vi "DNVideoX.vi"() -> ()   [LabVIEW 2015]
doc: "wdyjz@126.com\n完全访问USB cam， IP 网络照相机，TV tuner， DV 摄像机， PCI采集卡，fire-wire 或其他WDM兼容设备 \n支持多种视频输入"
panel:
  in  "Stop Capture":bool
  in  "StartCapture":bool
  in  "LEDOFF":bool
  in  "LED2":bool
  in  "LED1":bool
  in  "DNVideoX":refnum<k7>(container)
  out "Saved successfully":bool
  in  "Show Video Source Dialog":bool
  in  "Show Video Format Dialog":bool
  out "Camera count list":string[](array[string])
  out "Camera count":i32
  in  "Save Image":bool
  in  "氨ゎ":bool
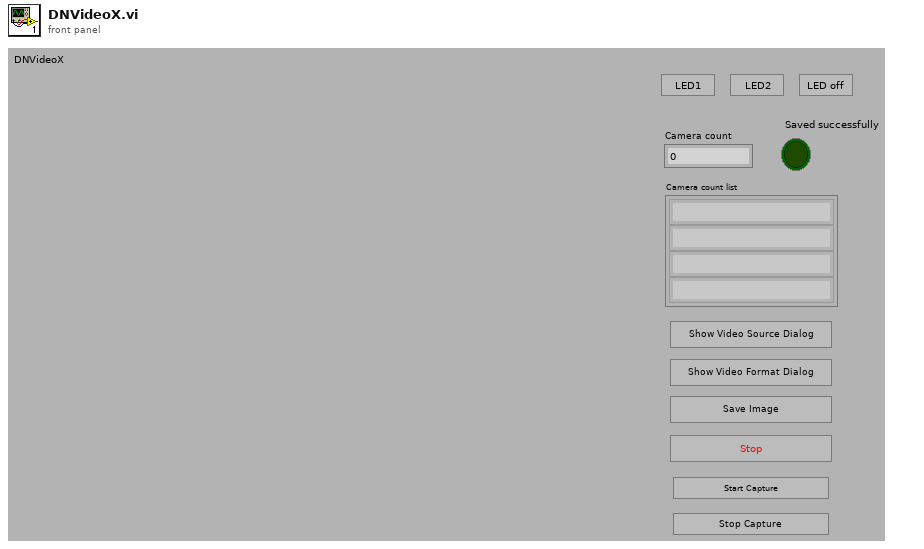
[diagram p1: front panel]
types:
  T1 = typedef "LVDateTimeRec.ctl" = cluster{"秒数的小数部分":dbl, "秒":i32, "分":i32, "小时":i32, "日":i32, "月":i32, "年":i32, "天数（周）":i32, "天数（年）":i32, "DST":i32}
  T2 = cluster{"秒数的小数部分":string, "秒":string, "分":string, "小时":string, "日":string, "月":string, "年":string, "天数（周）":string, "天数（年）":string, "DST":string}
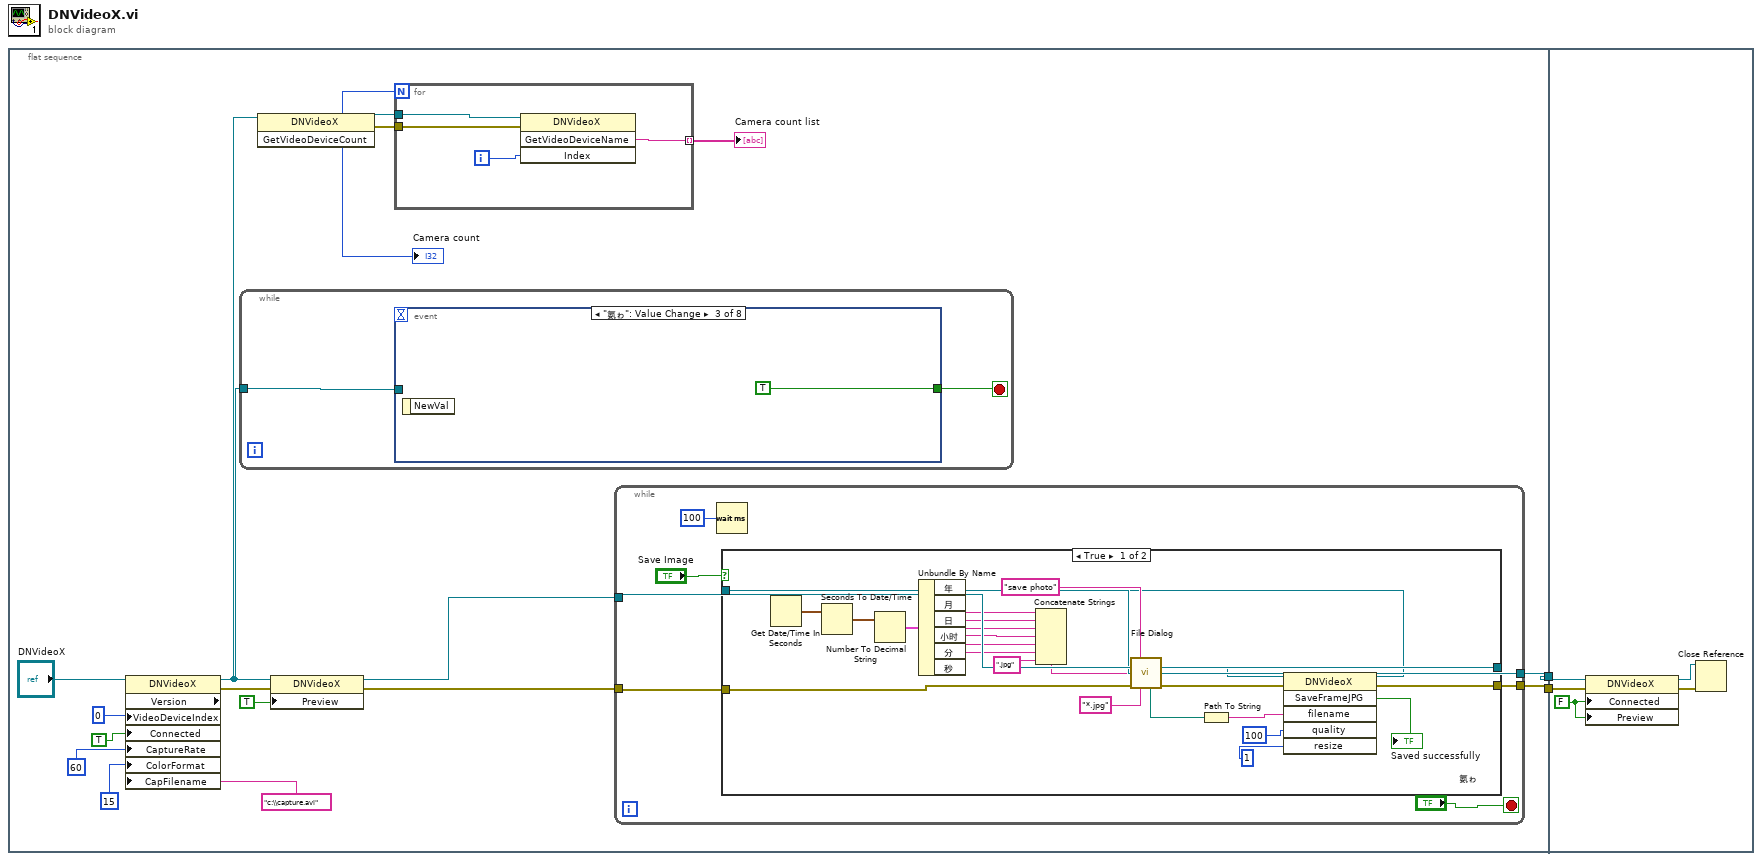
[diagram p0: block diagram]
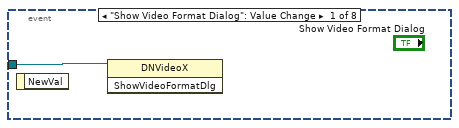
[diagram p2: hidden frame]
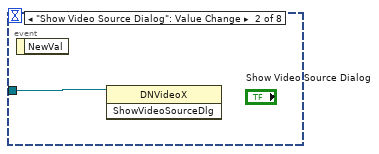
[diagram p3: hidden frame]
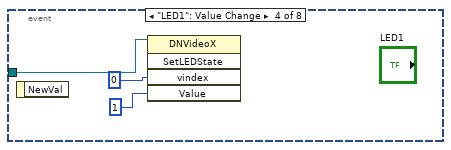
[diagram p4: hidden frame]
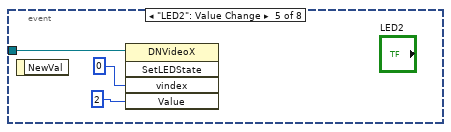
[diagram p5: hidden frame]
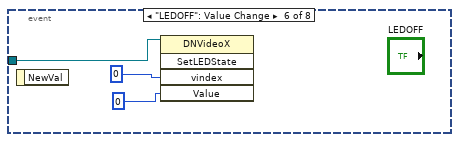
[diagram p6: hidden frame]
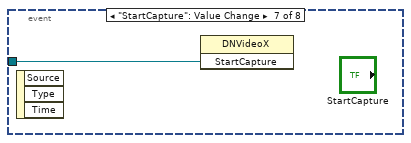
[diagram p7: hidden frame]
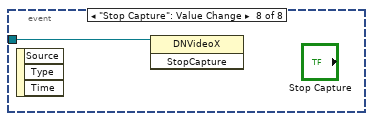
[diagram p8: hidden frame]
diagram:
  n1 = flat-sequence {
    tunnel: [w16] -> w2
    tunnel: [w9] -> w1
    tunnel: w2 -> [w76]
    tunnel: w1 -> [w72]
    frame #0 {
      n2 = property class="DNVideoX" props=["Version", "VideoDeviceIndex", "Connected", "CaptureRate", "ColorFormat", "CapFilename"](reference="DNVideoX", "VideoDeviceIndex"=0, "Connected"=TRUE, "CaptureRate"=60 ("VideoDeviceIndex"), "ColorFormat"=15 ("VideoDeviceIndex"), "CapFilename"="c:\\capture.avi" ("default name")) -> (reference out=w7:refnum<k7>, error out=w14:errorcluster)  [unwired: 1 in, 1 out]
      n3 = while {
        tunnel: w7 -> [w21]
        stop <- w20 stop-if-true
        n4 = event shown="[2] \"氨ゎ\": Value Change" {
          selector: _ -> [_ _ _ _ _ _ _ _]
          dyn-events: _ -> [_ _ _ _ _ _ _ _]
          timeout: _ -> [_ _ _ _ _ _ _ _]
          tunnel: w21 -> [w22 w23 _ w27 w30 w33 w34 w35]
          tunnel: [_ _ TRUE _ _ _ _ _] -> w20
          event "Show Video Format Dialog": Value Change {
            n5 = event-data() -> ()  [unwired: 2 out]
            n6 = invoke class="DNVideoX" method="ShowVideoFormatDlg"(reference=w22) -> ()  [unwired: 2 in, 3 out]
          }
          event "Show Video Source Dialog": Value Change {
            n7 = event-data() -> ()  [unwired: 2 out]
            n8 = invoke class="DNVideoX" method="ShowVideoSourceDlg"(reference=w23) -> ()  [unwired: 2 in, 3 out]
          }
          event "氨ゎ": Value Change {
            n9 = event-data() -> ()  [unwired: 2 out]
          }
          event "LED1": Value Change {
            n10 = event-data() -> ()  [unwired: 2 out]
            n11 = invoke class="DNVideoX" method="SetLEDState"(reference=w27, "vindex"=0, "Value"=1) -> ()  [unwired: 2 in, 5 out]
          }
          event "LED2": Value Change {
            n12 = event-data() -> ()  [unwired: 2 out]
            n13 = invoke class="DNVideoX" method="SetLEDState"(reference=w30, "vindex"=0, "Value"=2) -> ()  [unwired: 2 in, 5 out]
          }
          event "LEDOFF": Value Change {
            n14 = event-data() -> ()  [unwired: 2 out]
            n15 = invoke class="DNVideoX" method="SetLEDState"(reference=w33, "vindex"=0, "Value"=0) -> ()  [unwired: 2 in, 5 out]
          }
          event "StartCapture": Value Change {
            n16 = event-data() -> ()  [unwired: 4 out]
            n17 = invoke class="DNVideoX" method="StartCapture"(reference=w34) -> ()  [unwired: 2 in, 3 out]
          }
          event "Stop Capture": Value Change {
            n18 = event-data() -> ()  [unwired: 4 out]
            n19 = invoke class="DNVideoX" method="StopCapture"(reference=w35) -> ()  [unwired: 2 in, 3 out]
          }
        }
      }
      n20 = invoke class="DNVideoX" method="GetVideoDeviceCount"(reference=w7) -> (reference out=w10:refnum<k7>, error out=w12:errorcluster, "GetVideoDeviceCount"=w11:i32)  [unwired: 2 in]
      "Camera count" <- w11
      n21 = property class="DNVideoX"(reference=w7, error in=w14, "Preview"=TRUE) -> (reference out=w6:refnum<k7>, error out=w13:errorcluster)
      n22 = for {
        N: w11 -> [_]
        tunnel: [w36] -> w19 mode=indexing
        tunnel: w12 -> [w38]
        tunnel: w10 -> [w37]
        i -> [w39]
        n23 = invoke class="DNVideoX" method="GetVideoDeviceName"(reference=w37, error in=w38, "Index"=w39) -> ("GetVideoDeviceName"=w36:string)  [unwired: 1 in, 3 out]
      }
      "Camera count list" <- w19
      n24 = while {
        tunnel: w6 -> [w43]
        tunnel: [w42] -> w16
        tunnel: w13 -> [w41]
        tunnel: [w40] -> w9
        stop <- "氨ゎ" stop-if-true
        n25 = Wait (ms)(milliseconds to wait=u32 100 ("等待时间（毫秒）")) -> ()  [unwired: 1 out]
        n26 = case shown="True" "Save Image" {
          tunnel: w43 -> [w55 w71]
          tunnel: [w51 w71] -> w42
          tunnel: w41 -> [w50 w70]
          tunnel: [w48 w70] -> w40
          frame True {
            n27 = Get Date/Time In Seconds() -> (seconds since 1Jan1904=w58:timestamp)
            n28 = Seconds To Date/Time(time stamp (now)=w58) -> (date time rec=w57:T1)  [unwired: 1 out]
            n29 = Number To Decimal String(number=w57) -> (decimal integer string=w56:T2)  [unwired: 1 out]
            n30 = Unbundle By Name(w56) -> ("年"=w66:string, "月"=w65:string, "日"=w64:string, "小时"=w63:string, "分"=w62:string, "秒"=w61:string)
            n31 = Concatenate Strings(w66, w65, w64, w63, w62, w61, ".jpg" ("default name")) -> (w59:string)
            n32 = call "File Dialog"("prompt"="save photo", "default name"=w59, "error in"=w50, "pattern (all files)"="*.jpg") -> ("selected path"=w67:path, "error out"=w49:errorcluster)  [unwired: 3 in, 7 out]
            n33 = Path To String(path=w67) -> (string=w53:string)
            n34 = invoke class="DNVideoX" method="SaveFrameJPG"(reference=w55, error in=w49, "filename"=w53, "quality"=100, "resize"=1 ("quality")) -> (reference out=w51:refnum<k7>, error out=w48:errorcluster, "SaveFrameJPG"=→"Saved successfully":bool)  [unwired: 1 in, 3 out]
          }
          frame False {
          }
        }
      }
    }
    frame #1 {
      w75 = FALSE ("Connected")
      n35 = property class="DNVideoX"(reference=w76, error in=w72, "Connected"=w75, "Preview"=w75) -> (reference out=w74:refnum<k7>, error out=w73:errorcluster)
      n36 = Close Reference(reference=w74, error in (no error)=w73) -> ()  [unwired: 1 out]
    }
  }
